vi "Write FitControlToPane Option.vi"(8 "error in (no error)":errorcluster, 10 "FitControlToPane Option":bool, 11 "AdjustableMulticolumnListbox in":refnum<class "AdjMCLB.lvclass">) -> (0 "error out":errorcluster, 3 "AdjustableMulticolumnListbox out":refnum<class "AdjMCLB.lvclass">)   [LabVIEW 2020, in "AdjMCLB.lvclass"]
uses:
  AdjMCLB.lvclass
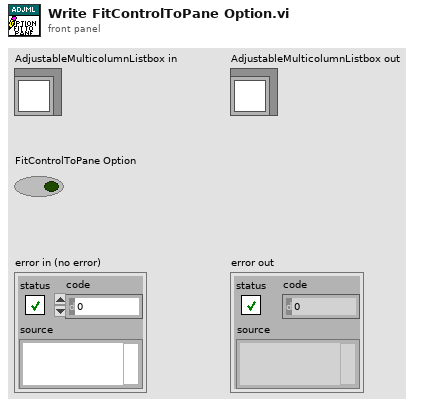
[diagram p1: front panel]
types:
  T1 = typedef "AdjustableMulticolumnListbox.lvclass/State Data.ctl" = cluster{"FitControlToPane?":bool, "ColumnSizes":i32[]}
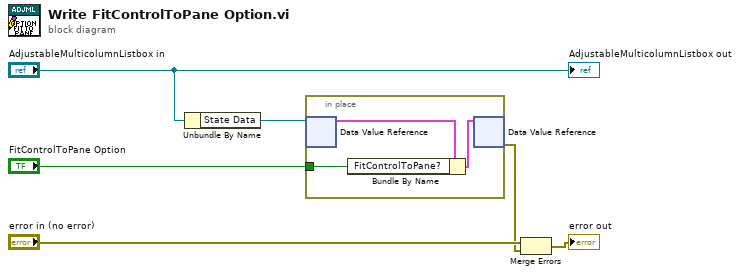
[diagram p0: block diagram]
diagram:
  n1 = Unbundle By Name("AdjustableMulticolumnListbox in") -> ("State Data"=w4:refnum<data-value>)
  n2 = in-place {
    in-place-border: "FitControlToPane Option" -> [w7]
    n3 = in-place-dvr #1(w4) -> (w9:T1)  [unwired: 1 out]
    n4 = Bundle By Name(cluster=w9, "FitControlToPane?"=w7) -> (w8:T1)
    n5 = in-place-dvr #1(w8) -> (w1:errorcluster)  [unwired: 1 out]
  }
  n6 = Merge Errors("error in (no error)", w1) -> (→"error out":errorcluster)
  "AdjustableMulticolumnListbox out" <- "AdjustableMulticolumnListbox in"
